vi "2-13.vi"() -> ()   [LabVIEW 2022 SP3]
panel:
  out "实时温度:":dbl format="%#_4f"
  in  "ON":bool
  out "运行时间(s):":dbl
  in  "采集时间(s)":dbl(knob) scale=0.0..3.0 scale format="%#_4g"
  out "温度实时曲线":dbl(graph)
  # "OFF"
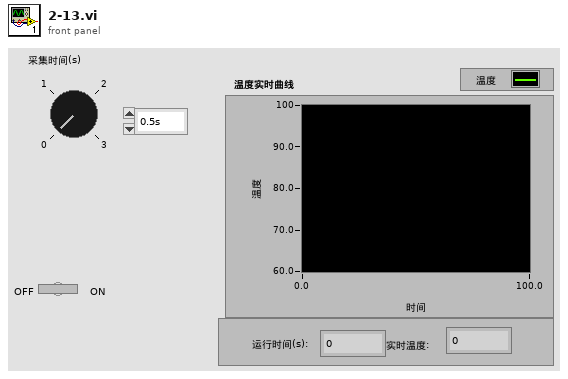
[diagram p1: front panel]
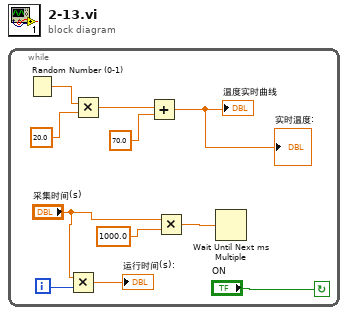
[diagram p0: block diagram]
diagram:
  n1 = while {
    i -> [w4]
    stop <- "ON" continue-if-true
    n2 = Random Number (0-1)() -> (number: 0 to 1=w10:dbl)
    n3 = Multiply(x="采集时间(s)", y=w4) -> (x*y=→"运行时间(s):":dbl)
    n4 = Multiply(x=w10, y=20.0) -> (x*y=w8:dbl)
    n5 = Add(x=w8, y=70.0) -> (x+y=→"温度实时曲线" →"实时温度:":dbl)
    n6 = Multiply(x="采集时间(s)", y=1000.0) -> (x*y=w5:dbl)
    n7 = Wait Until Next ms Multiple(millisecond multiple=w5) -> ()  [unwired: 1 out]
  }
